vi "Menu Button - Update Header.vi"(11 "Display State In in":T1={"Header"="", "Label[]"=[], "DisableButtonsLUT"=variant(string[] []), "Menu Config"=variant}) -> (2 "Header":string, 3 "Display State In out":T1={"Header"="", "Label[]"=[], "DisableButtonsLUT"=variant(string[] []), "Menu Config"=variant})   [LabVIEW 2019, in "Menu Button.xctl"]
doc: "JSMA Module Template - Top Level UI 0.2.0.4\nRob Humfeld - Jet Engineering\nCopyright (c) 2019, Jet Engineering"
uses:
  Menu Button.xctl
  State 1.ctl
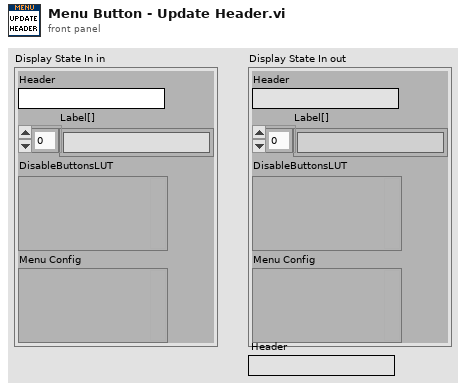
[diagram p1: front panel]
types:
  T1 = typedef "Menu Button.xctl/State 1.ctl" = cluster{"Header":string, "Label[]":string[], "DisableButtonsLUT":variant, "Menu Config":variant}
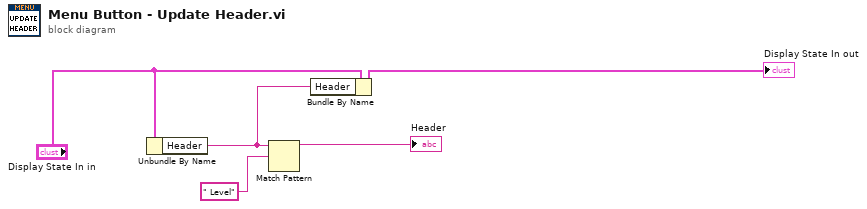
[diagram p0: block diagram]
diagram:
  n1 = Unbundle By Name("Display State In in") -> ("Header"=w5:string)
  n2 = Match Pattern(string=w5, regular expression=" Level") -> (before substring=→"Header":string)  [unwired: 1 in, 3 out]
  n3 = Bundle By Name(cluster="Display State In in", "Header"=w5) -> (→"Display State In out":T1)
